vi "VisionInit.vi"(8 "error in (no error)":errorcluster, 11 "Refnum in":T2) -> (0 "error out":errorcluster, 2 "New Image":T1, 3 "Refnum out":T2)   [LabVIEW 2021]
uses:
  <vilib>/userDefined/High Color/IMAQdx.ctl
  <vilib>/vision/Image Controls.llb/IMAQ Image.ctl
  <vilib>/vision/driver/IMAQdx.llb/IMAQdx Acquisition Mode.ctl
  <vilib>/vision/driver/NI_Vision_Acquisition_Software.lvlib
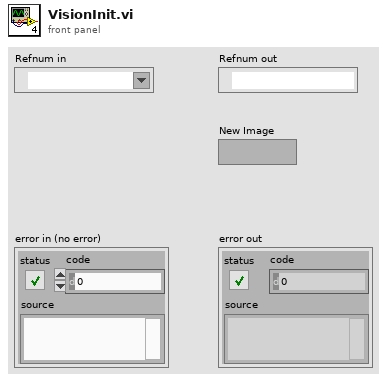
[diagram p1: front panel]
types:
  T1 = typedef "IMAQ Image.ctl" = refnum<image>
  T2 = typedef "IMAQdx.ctl" = refnum<k21>
  T3 = typedef "Image Type" = u32
  T4 = typedef "NI_Vision_Acquisition_Software.lvlib/IMAQdx Acquisition Mode.ctl" = enum32{"One Shot", "Continuous"}
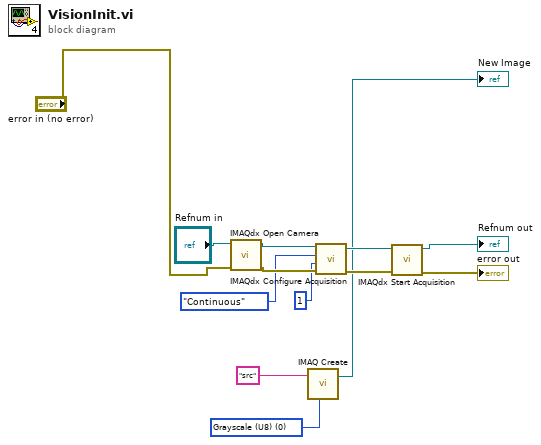
[diagram p0: block diagram]
diagram:
  w2 = T3 0 items=["Grayscale (U8)", "Grayscale (I16)", "Grayscale (SGL)", "Complex (CSG)", "RGB (U32)", "HSL (U32)", "RGB (U64)", "Grayscale (U16)"] ("Image Type")
  n1 = call <vilib>:"IMAQdx Open Camera.vi"("error in"="error in (no error)", "Session In"="Refnum in") -> ("error out"=w7:errorcluster, "Session Out"=w8:T2)  [unwired: 8 in]
  n2 = call "IMAQ Create"("Image Name"="src", "Image Type"=w2) -> ("New Image"=→"New Image":T1)  [unwired: 3 in, 1 out]
  n3 = call <vilib>:"IMAQdx Configure Acquisition.vi"("error in"=w7, "Number of Buffers"=u32 1, "Continuous?"=IMAQdx_Acquisition_Mode."Continuous", "Session In"=w8) -> ("error out"=w12:errorcluster, "Session Out"=w11:T2)  [unwired: 6 in]
  n4 = call <vilib>:"IMAQdx Start Acquisition.vi"("error in"=w12, "Session In"=w11) -> ("error out"=→"error out":errorcluster, "Session Out"=→"Refnum out":T2)  [unwired: 8 in]
